vi "newBookingEmail.vi"(4 "device name":string, 5 "email sender":string="cuallita202@yahoo.es", 6 "smtp server":string, 7 "recipients":string[](array[string]), 8 "email student":string) -> (0 "error out":errorcluster)   [LabVIEW 2010]
uses:
  <vilib>/Utility/SMTP/NI_SMTPEmail.lvlib
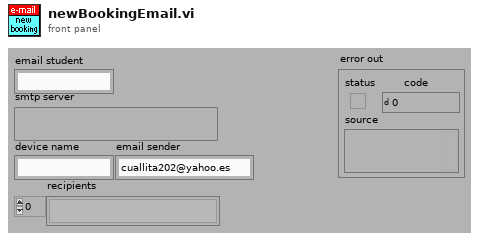
[diagram p1: front panel]
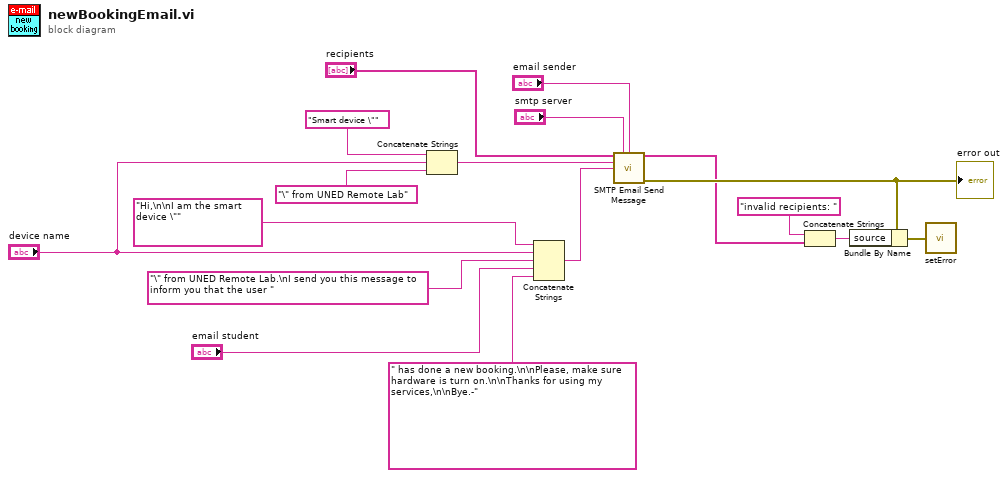
[diagram p0: block diagram]
diagram:
  n1 = Concatenate Strings("Smart device \"" ("subject ([No Subject])"), "device name", "\" from UNED Remote Lab" ("subject ([No Subject])")) -> (w2:string)
  n2 = Concatenate Strings("Hi,\n\nI am the smart device \"" ("Connection report"), "device name", "\" from UNED Remote Lab.\nI send you this message to inform you that the user " ("Connection report"), "email student", " has done a new booking.\n\nPlease, make sure hardware is turn on.\n\nThanks for using my services,\n\nBye.-" ("Connection report")) -> (w15:string)
  n3 = call <vilib>:"SMTP Email Send Message.vi"("recipients"="recipients", "mail server"="smtp server", "return address"="email sender", "subject ([No Subject])"=w2, "message"=w15) -> ("invalid recipients"=w8:string[], "error out"=w11:errorcluster)  [unwired: 1 in, 8 out]
  "error out" <- w11
  n4 = Concatenate Strings("invalid recipients: " ("string"), w8) -> (w7:string)
  n5 = Bundle By Name(cluster=w11, "source"=w7) -> (w10:errorcluster)
  n6 = call "setError.vi"("error"=w10) -> ()  [unwired: 1 out]
